vi "Subvi AO.vi"(2 "AO":refnum<k21>="Connector1/AO0", 8 "Manual trigger":bool, 10 "FIFO In":refnum<k21>="AB0") -> ()   [LabVIEW 2017]
uses:
  <vilib>/rvi/DataTransferAndStorage/Container/XNode/niFpgaContainer.xnode
  <vilib>/rvi/FIFO/Fifo_Resource/niFpgaFifoEmulationRefIn.vi
  GV FIFO timeout.vi
  <vilib>/eio/EIONode/EIONode.xnode
  <vilib>/rvi/eio/common/nirviEmuTemplateMethod_errors.vi
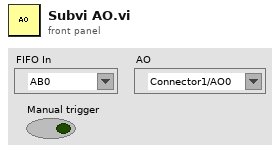
[diagram p1: front panel]
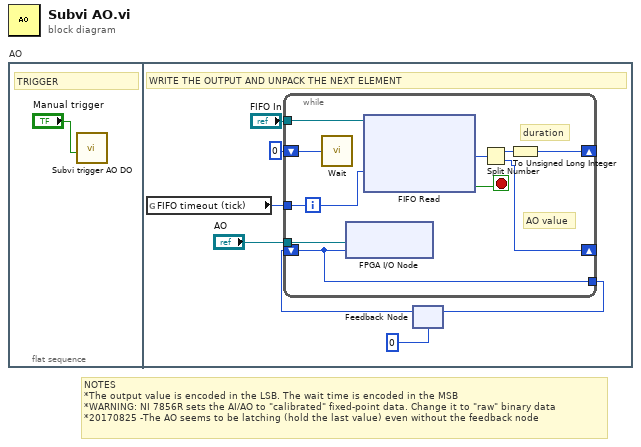
[diagram p0: block diagram]
diagram:
  # "NOTES\n*The output value is encoded in the LSB. The wait time is encoded in the MSB\n*WARNING: NI 7856R sets the AI/AO to \"calibrated\" fixed-point data. Change it to \"raw\" binary data\n*20170825 -The AO seems to be latching (hold the last value) even without the feedback node"
  n1 = flat-sequence "AO" {
    frame #0 {
      # "TRIGGER"
      n2 = call "Subvi trigger AO DO.vi"("Manual trigger"="Manual trigger") -> ()  [unwired: 11 in]
    }
    frame #1 {
      # "WRITE THE OUTPUT AND UNPACK THE NEXT ELEMENT"
      n3 = global read "GV FIFO timeout.vi" "FIFO timeout (tick)"() -> (w4:i32)
      n4 = feedback #1(u16 0) -> (w7:u16)
      n5 = while {
        shift-right: [w11] -> _
        shift-left: u32 0 -> [w18]
        shift-right: [w16] -> _
        shift-left: w7 -> [w9]
        tunnel: [w9] -> w5
        tunnel: "FIFO In" -> [w13]
        tunnel: w4 -> [w12]
        tunnel: "AO" -> [w10]
        stop <- w14 stop-if-true
        # "duration"
        # "AO value"
        n6 = call "Wait"("Count(Ticks)"=w18) -> ()  [unwired: 1 out]
        n7 = xnode "FPGA I/O Node"("I/O Item"=w9, "FPGA I/O In"=w10) -> ()  [unwired: 1 out]
        n8 = xnode ("FIFO Read")("Timeout"=w12, "FIFO In"=w13) -> ("Element"=w15:u32, "Timed Out?"=w14:bool)  [unwired: 1 out]
        n9 = Split Number(x=w15) -> (hi(x)=w17:u16, lo(x)=w16:u16)
        n10 = To Unsigned Long Integer(number=w17) -> (unsigned 32bit integer=w11:u32)
      }
      n11 = feedback-in #1(w5) -> ()
    }
  }
